vi "SIM Registry Update Header Field.vi"(8 "New Value":i32, 9 "Field":T1, 10 "Block Idx":i32, 11 "Node Headers":T2[](array[typedef])) -> (2 "Block Idx Out":i32, 3 "Node Headers Out":T2[](array[typedef]))   [LabVIEW 2017]
uses:
  <vilib>/Simulation/Implementation/Shared/SIM Registry.llb/SIM Registry Node Header.ctl
  <vilib>/Simulation/Implementation/Shared/SIM Registry.llb/SIM Registry Header Fields.ctl
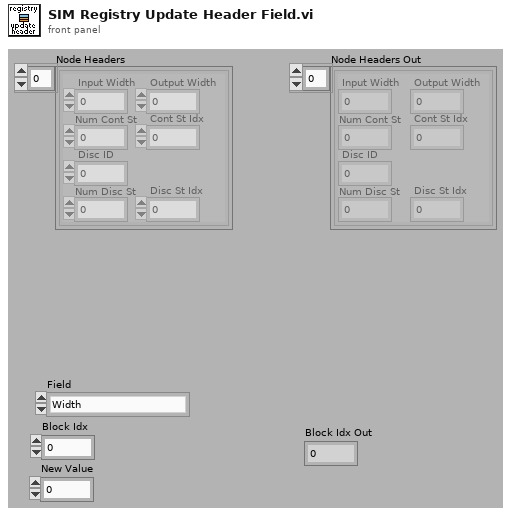
[diagram p1: front panel]
types:
  T1 = typedef "SIM Registry Header Fields.ctl" = enum16{"Width", "Disc ID", "Num States", "State Idx", "Num Disc States", "Disc State Idx"}
  T2 = typedef "SIM Registry Node Header.ctl" = cluster{"Input Width":i32, "Disc ID":i32, "Num Cont St":i32, "Cont St Idx":i32, "Num Disc St":i32, "Disc St Idx":i32, "Output Width":i32}
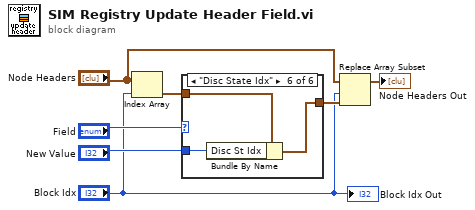
[diagram p0: block diagram]
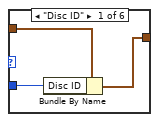
[diagram p2: hidden frame]
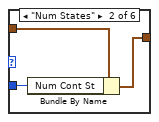
[diagram p3: hidden frame]
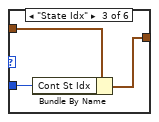
[diagram p4: hidden frame]
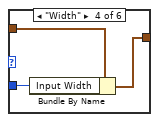
[diagram p5: hidden frame]
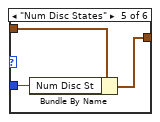
[diagram p6: hidden frame]
diagram:
  n1 = Index Array(array="Node Headers", index="Block Idx") -> (element=w4:T2)
  n2 = case shown="\"Disc State Idx\"" "Field" {
    tunnel: w4 -> [w10 w13 w16 w19 w22 w25]
    tunnel: "New Value" -> [w9 w12 w15 w18 w21 w24]
    tunnel: [w8 w11 w14 w17 w20 w23] -> w5
    frame "Disc ID" {
      n3 = Bundle By Name(cluster=w10, "Disc ID"=w9) -> (w8:T2)
    }
    frame "Num States" {
      n4 = Bundle By Name(cluster=w13, "Num Cont St"=w12) -> (w11:T2)
    }
    frame "State Idx" {
      n5 = Bundle By Name(cluster=w16, "Cont St Idx"=w15) -> (w14:T2)
    }
    frame "Width" {
      n6 = Bundle By Name(cluster=w19, "Input Width"=w18) -> (w17:T2)
    }
    frame "Num Disc States" {
      n7 = Bundle By Name(cluster=w22, "Num Disc St"=w21) -> (w20:T2)
    }
    frame "Disc State Idx" {
      n8 = Bundle By Name(cluster=w25, "Disc St Idx"=w24) -> (w23:T2)
    }
  }
  n9 = Replace Array Subset(array="Node Headers", new element=w5, index="Block Idx") -> (→"Node Headers Out":T2[])
  "Block Idx Out" <- "Block Idx"
